vi "Recognize Gesture.vi"(11 "mouse":T1) -> (3 "gesture":refnum<class "Gesture.lvclass">)   [LabVIEW 2019, in "Gesture.lvclass"]
doc: "Determine the state of the gesture based on current and previous state, start time, and mouse position."
uses:
  Gesture.lvclass
  <vilib>/Utility/miscctls.llb/LVMouseTypeDef.ctl
  Recognize Gesture State.ctl
  Gesture Enum.ctl
panel:
  # "option drag up is pinch open\noption drag down is pinch close"
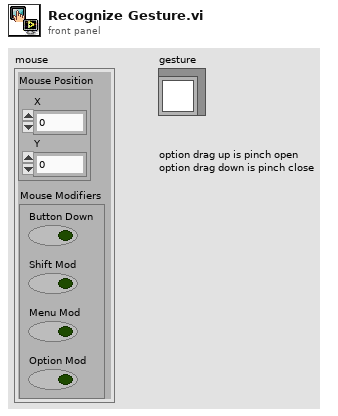
[diagram p1: front panel]
types:
  T1 = typedef "LVMouseTypeDef.ctl" = cluster{"Mouse Position":cluster{"X":i32, "Y":i32}, "Mouse Modifiers":cluster{"Button Down":bool, "Shift Mod":bool, "Menu Mod":bool, "Option Mod":bool}}
  T2 = typedef "GestureRecognizerState.ctl" = enum16{"idle", "start", "press", "panning", "pinch", "tap"}
  T3 = typedef "Gesture.lvclass/Recognize Gesture State.ctl" = enum16{"idle", "start", "press", "panning", "pinch", "tap"}
  T4 = typedef "Gesture.lvclass/Gesture Enum.ctl" = enum16{"None", "Stop", "Tap", "Press", "Pan Start", "Pan Continue", "Pan End", "Pinch Open", "Pinch Close", "Double Tap"}
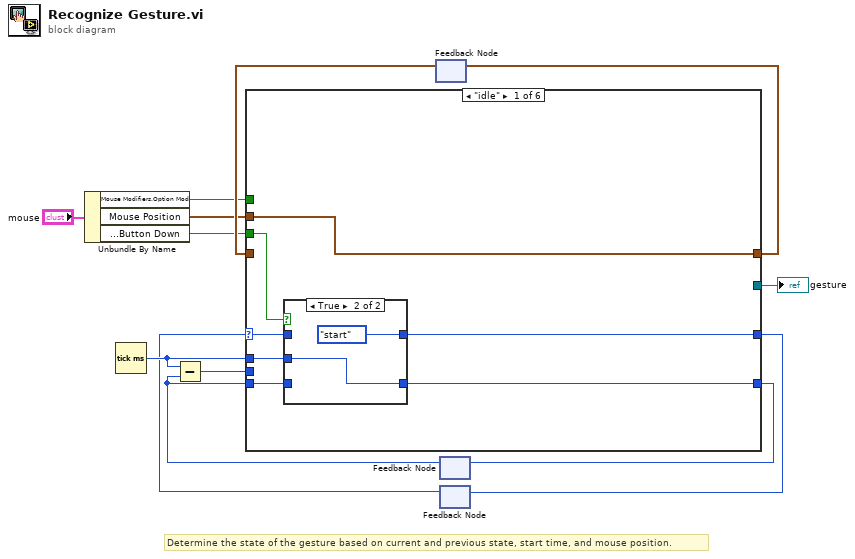
[diagram p0: block diagram]
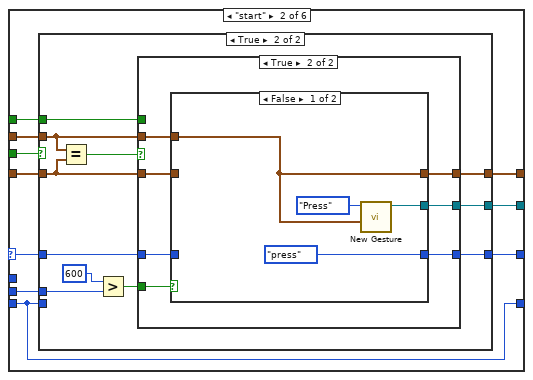
[diagram p3: hidden frame]
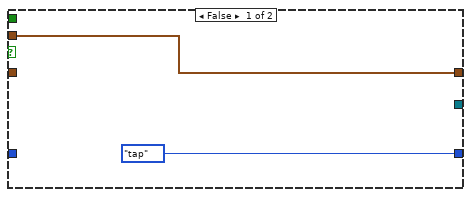
[diagram p4: hidden frame]
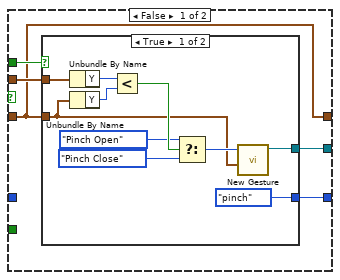
[diagram p5: hidden frame]
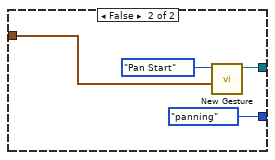
[diagram p6: hidden frame]
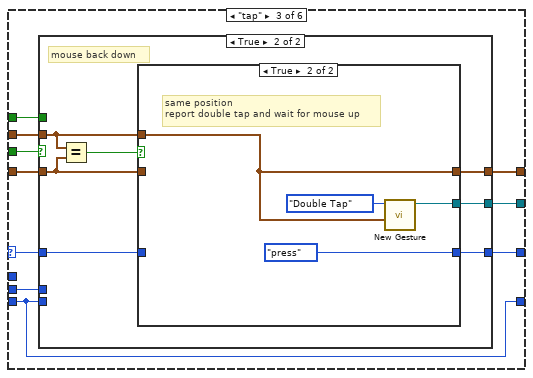
[diagram p8: hidden frame]
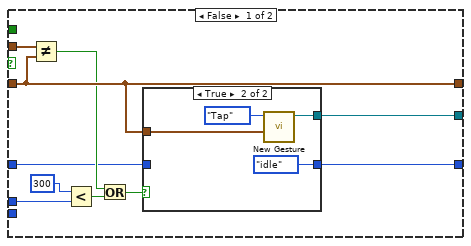
[diagram p9: hidden frame]
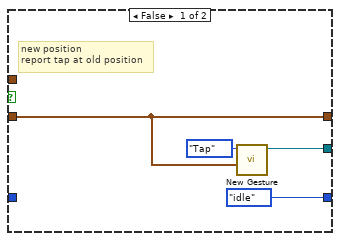
[diagram p11: hidden frame]
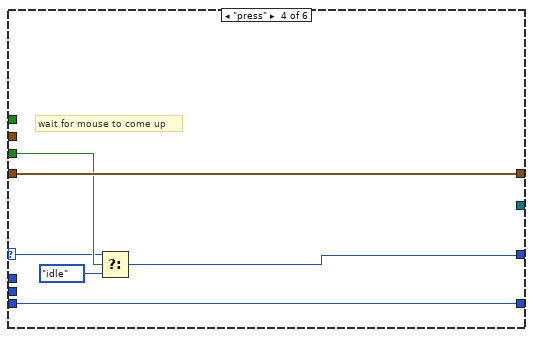
[diagram p12: hidden frame]
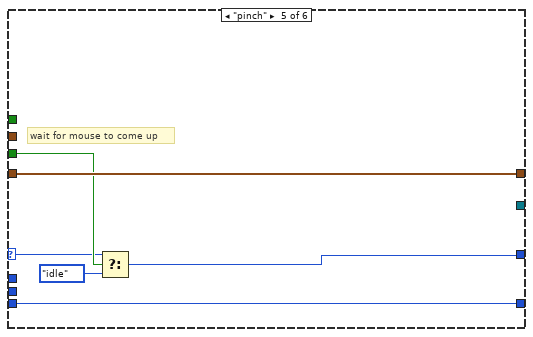
[diagram p13: hidden frame]
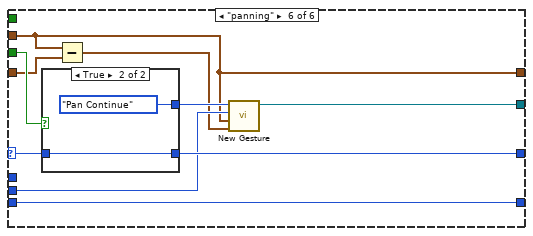
[diagram p14: hidden frame]
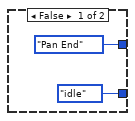
[diagram p15: hidden frame]
diagram:
  # "Determine the state of the gesture based on current and previous state, start time, and mouse position."
  n1 = Unbundle By Name("mouse") -> ("Mouse Modifiers.Option Mod"=w4:bool, "Mouse Position"=w5:cluster{"X":i32, "Y":i32}, "Mouse Modifiers.Button Down"=w6:bool)
  n2 = Tick Count (ms)() -> (millisecond timer value=w3:u32)
  n3 = feedback #1() -> (w10:cluster{"X":i32, "Y":i32})  [unwired: 1 in]
  n4 = feedback #2() -> (w8:u32)  [unwired: 1 in]
  n5 = Subtract(x=w3, y=w8) -> (x-y=w2:u32)
  n6 = feedback #3() -> (w1:T2)  [unwired: 1 in]
  n7 = case shown="\"idle\"" w1 {
    selector: w1 -> [w17 w28 w83 w121 w126 w139]
    tunnel: w6 -> [w19 w34 w89 w123 w129 w141]
    tunnel: [w14 w30 w85 w120 w128 w140] -> w7
    tunnel: [_ w33 w88 _ _ w137] -> w12
    tunnel: [w18 w25 w80 w124 w130 w138] -> w9
    tunnel: w8 -> [w16 w25 w80 w124 w130 w138]
    tunnel: [w20 w29 w84 w125 w131 w132] -> w11
    tunnel: w5 -> [w20 w31 w86 _ _ w132]
    tunnel: w10 -> [_ w32 w87 w125 w131 w134]
    tunnel: w4 -> [_ w27 w82 _ _ _]
    tunnel: w2 -> [_ w26 w81 _ _ w136]
    tunnel: w3 -> [w15 _ _ _ _ _]
    frame "idle" {
      n8 = case shown="True" w19 {
        tunnel: [w22 Recognize_Gesture_State."start" ("t")] -> w14
        tunnel: [w21 w23] -> w18
        tunnel: w17 -> [w22 _]
        tunnel: w16 -> [w21 _]
        tunnel: w15 -> [_ w23]
        frame False {
        }
        frame True {
        }
      }
    }
    frame "start" {
      n9 = case shown="True" w34 {
        tunnel: [Recognize_Gesture_State."tap" ("state") w45] -> w30
        tunnel: [_ w46] -> w33
        tunnel: w25 -> [_ _]
        tunnel: w32 -> [_ w43]
        tunnel: w31 -> [w36 w44]
        tunnel: w28 -> [_ w42]
        tunnel: [w36 w41] -> w29
        tunnel: w27 -> [_ w38]
        tunnel: w26 -> [_ w37]
        frame False {
        }
        frame True {
          n10 = Equal?(x=w44, y=w43) -> (x = y?=w40:bool)
          n11 = Greater?(x=u32 600 ("y"), y=w37) -> (0:w39:bool)
          n12 = case shown="True" w40 {
            tunnel: [w51 w73] -> w46
            tunnel: [w52 w72] -> w45
            tunnel: w44 -> [w49 w71]
            tunnel: w43 -> [w48 w68]
            tunnel: w42 -> [_ w67]
            tunnel: [w48 w69] -> w41
            tunnel: w39 -> [_ w70]
            tunnel: w38 -> [w50 _]
            frame False {
              n13 = case shown="True" w50 {
                tunnel: [Recognize_Gesture_State."pinch" ("state") Recognize_Gesture_State."panning" ("state")] -> w52
                tunnel: [w55 w65] -> w51
                tunnel: w48 -> [w53 w63]
                tunnel: w49 -> [w61 _]
                frame True {
                  n14 = Unbundle By Name(w61) -> ("Y"=w60:i32)
                  n15 = Unbundle By Name(w53) -> ("Y"=w59:i32)
                  n16 = Less?(x=w60, y=w59) -> (x < y?=w58:bool)
                  n17 = Select(t=Gesture_Enum."Pinch Open" ("gesture"), s=w58, f=Gesture_Enum."Pinch Close" ("gesture")) -> (s? t:f=w54:T4)
                  n18 = call "New Gesture.vi"("point"=w53, "gesture"=w54) -> ("gesture out"=w55:refnum<class "Gesture.lvclass">)  [unwired: 9 in]
                }
                frame False {
                  n19 = call "New Gesture.vi"("point"=w63, "gesture"=Gesture_Enum."Pan Start") -> ("gesture out"=w65:refnum<class "Gesture.lvclass">)  [unwired: 9 in]
                }
              }
            }
            frame True {
              n20 = case shown="False" w70 {
                tunnel: [w74 _] -> w73
                tunnel: [Recognize_Gesture_State."press" ("state") w78] -> w72
                tunnel: w71 -> [w75 _]
                tunnel: [w75 w79] -> w69
                tunnel: w68 -> [_ w79]
                tunnel: w67 -> [_ w78]
                frame False {
                  n21 = call "New Gesture.vi"("point"=w75, "gesture"=Gesture_Enum."Press") -> ("gesture out"=w74:refnum<class "Gesture.lvclass">)  [unwired: 9 in]
                }
                frame True {
                }
              }
            }
          }
        }
      }
    }
    frame "tap" {
      n22 = case shown="True" w89 {
        tunnel: [w98 w110] -> w85
        tunnel: [w99 w111] -> w88
        tunnel: w80 -> [_ _]
        tunnel: w87 -> [w92 w108]
        tunnel: w86 -> [w93 w109]
        tunnel: w83 -> [w90 w107]
        tunnel: [w92 w106] -> w84
        tunnel: w82 -> [_ _]
        tunnel: w81 -> [w96 _]
        frame False {
          n23 = Not Equal?(x=w93, y=w92) -> (x != y?=w91:bool)
          n24 = Less?(x=u32 300 ("y"), y=w96) -> (x < y?=w95:bool)
          n25 = Or(x=w91, y=w95) -> (x .or. y?=w94:bool)
          n26 = case shown="True" w94 {
            tunnel: [_ w103] -> w99
            tunnel: [w100 Recognize_Gesture_State."idle" ("state")] -> w98
            tunnel: w92 -> [_ w102]
            tunnel: w90 -> [w100 _]
            frame False {
            }
            frame True {
              n27 = call "New Gesture.vi"("point"=w102, "gesture"=Gesture_Enum."Tap") -> ("gesture out"=w103:refnum<class "Gesture.lvclass">)  [unwired: 9 in]
            }
          }
        }
        frame True {
          # "mouse back down"
          n28 = Equal?(x=w109, y=w108) -> (x = y?=w105:bool)
          n29 = case shown="True" w105 {
            tunnel: [w114 w118] -> w111
            tunnel: [Recognize_Gesture_State."idle" ("state") Recognize_Gesture_State."press" ("state")] -> w110
            tunnel: w109 -> [_ w117]
            tunnel: w108 -> [w112 _]
            tunnel: w107 -> [_ _]
            tunnel: [w112 w117] -> w106
            frame False {
              # "new position\nreport tap at old position"
              n30 = call "New Gesture.vi"("point"=w112, "gesture"=Gesture_Enum."Tap") -> ("gesture out"=w114:refnum<class "Gesture.lvclass">)  [unwired: 9 in]
            }
            frame True {
              # "same position\nreport double tap and wait for mouse up"
              n31 = call "New Gesture.vi"("point"=w117, "gesture"=Gesture_Enum."Double Tap") -> ("gesture out"=w118:refnum<class "Gesture.lvclass">)  [unwired: 9 in]
            }
          }
        }
      }
    }
    frame "press" {
      # "wait for mouse to come up"
      n32 = Select(t=w121, s=w123, f=Recognize_Gesture_State."idle") -> (s? t:f=w120:T3)
    }
    frame "pinch" {
      # "wait for mouse to come up"
      n33 = Select(t=w126, s=w129, f=Recognize_Gesture_State."idle") -> (s? t:f=w128:T3)
    }
    frame "panning" {
      n34 = case shown="True" w141 {
        tunnel: [Recognize_Gesture_State."idle" ("state") w145] -> w140
        tunnel: w139 -> [_ w145]
        tunnel: [Gesture_Enum."Pan End" ("gesture") Gesture_Enum."Pan Continue" ("gesture")] -> w135
        frame False {
        }
        frame True {
        }
      }
      n35 = Subtract(x=w132, y=w134) -> (x-y=w133:cluster{"X":i32, "Y":i32})
      n36 = call "New Gesture.vi"("offset"=w133, "point"=w132, "elapsed time"=w136, "gesture"=w135) -> ("gesture out"=w137:refnum<class "Gesture.lvclass">)  [unwired: 7 in]
    }
  }
  "gesture" <- w12
  n37 = feedback-in #1(w11) -> ()
  n38 = feedback-in #2(w9) -> ()
  n39 = feedback-in #3(w7) -> ()
